vi "CRYUpdate Repeat State.vi"(0 "destination Index1":i32, 1 "fOption":bool, 5 "destination Index2":i32, 7 "My Index":i32, 9 "Start":dbl format="%#_5g", 11 "Increment":dbl, 12 "Count":i32, 13 "VI No":i32) -> (4 "fResult":bool)   [LabVIEW 2013]
uses:
  CRYProject Editor Global.vi
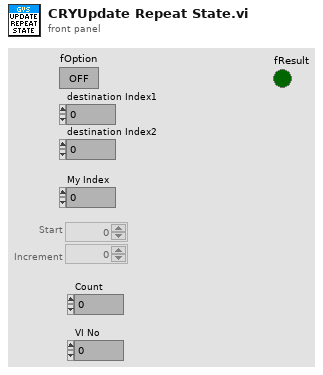
[diagram p1: front panel]
types:
  T1 = enum16{"OK", "Yes", "YesNo", "YesNoCancel", "ReplaceAppend"}
  T2 = typedef "CRYTS.ctl" = cluster{"No.TS":u16, "TS File Path":path, "TS Name":string, "EditStepName":string, "Steps":T3[], "New State":bool, "Change State":bool, "Flattened CurveLib Data":string, "Document Data":string, "EditStepNo":u16, "Operator Start File":string, "Sequence Type":string, "Sequence Language":string}
  T3 = typedef "CRYStep.ctl" = cluster{"No.VI":i32, "Category":string, "StepName":string, "Seq setup flattened":string, "Comment":string, "Steps config.":bool[], "Jump config":i32[], "Start":dbl, "Increment":dbl, "Name":string, "Unit":string, "Y data":u16, "Y prefix":string, "Y dB ref":dbl, "Y unit":string, "Repeat State Array":cluster{"Start":dbl, "Increment":dbl, "Count":i32, "Num":i32}[]}
  T4 = cluster{"Start":dbl, "Increment":dbl, "Count":i32, "Num":i32}[]
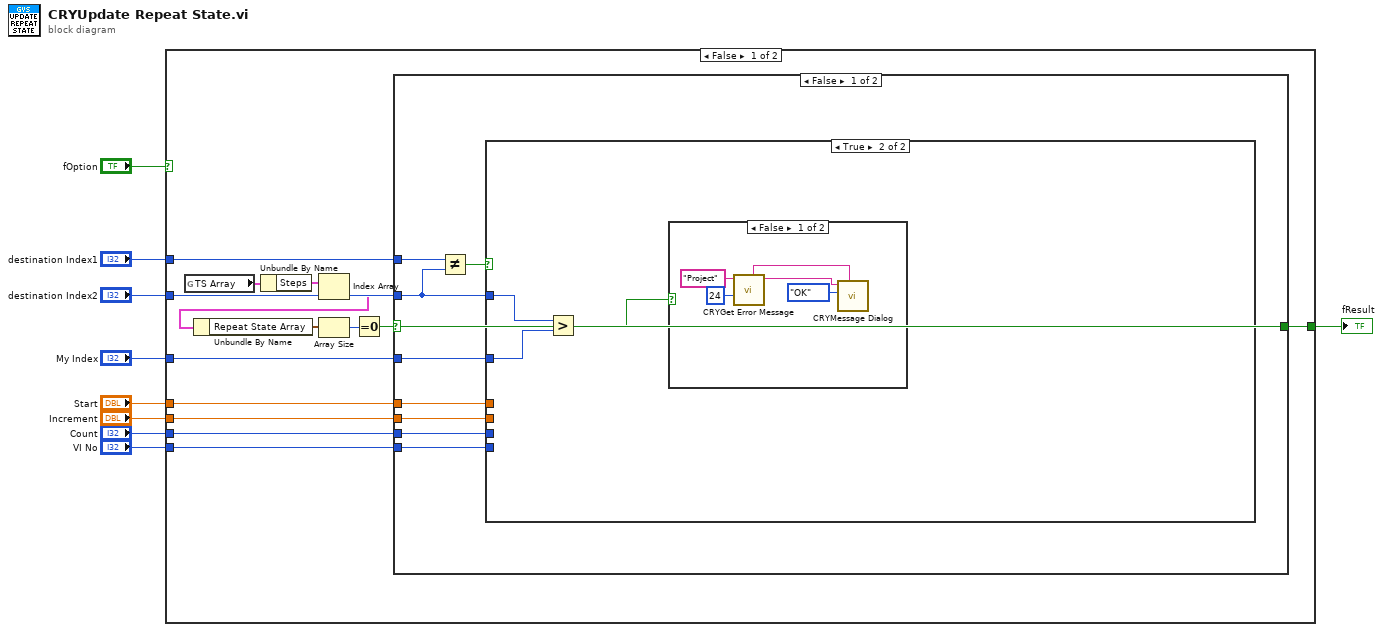
[diagram p0: block diagram]
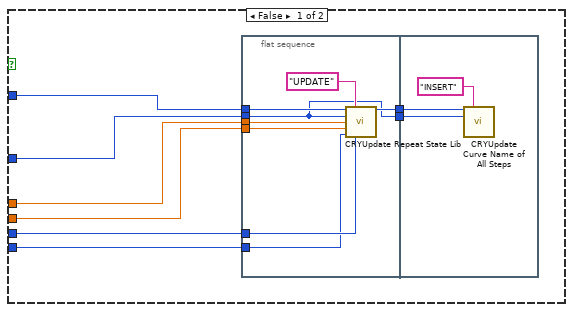
[diagram p2: hidden frame]
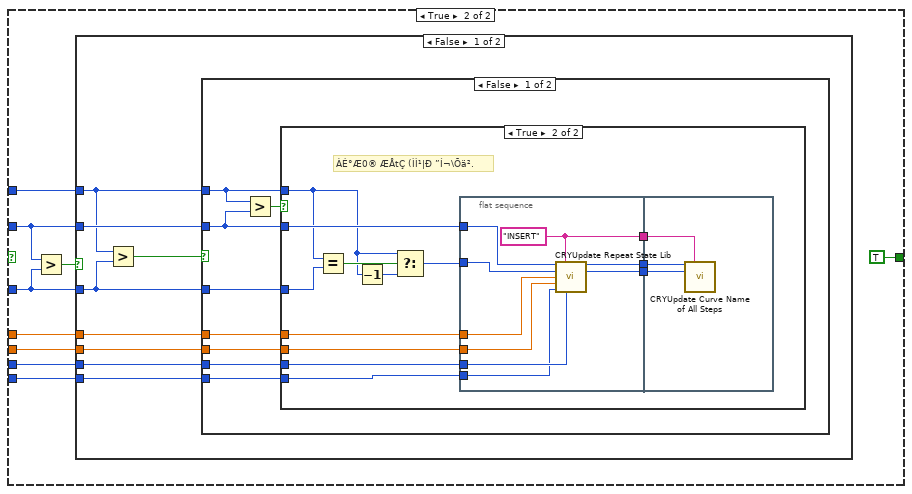
[diagram p4: hidden frame]
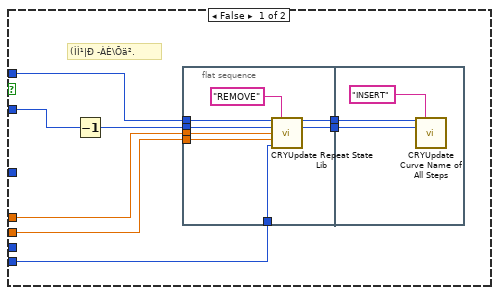
[diagram p5: hidden frame]
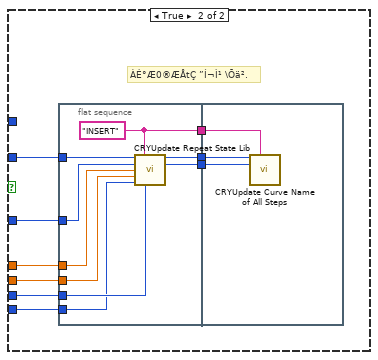
[diagram p6: hidden frame]
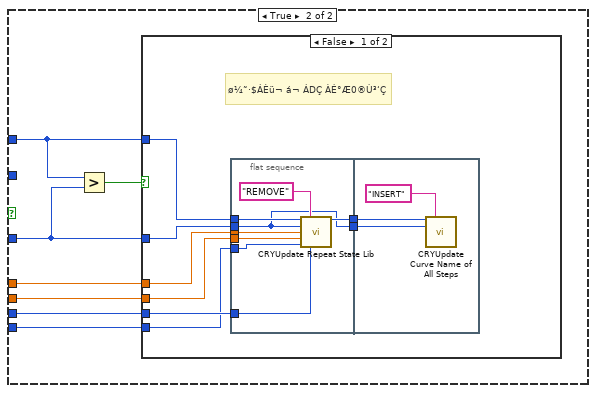
[diagram p7: hidden frame]
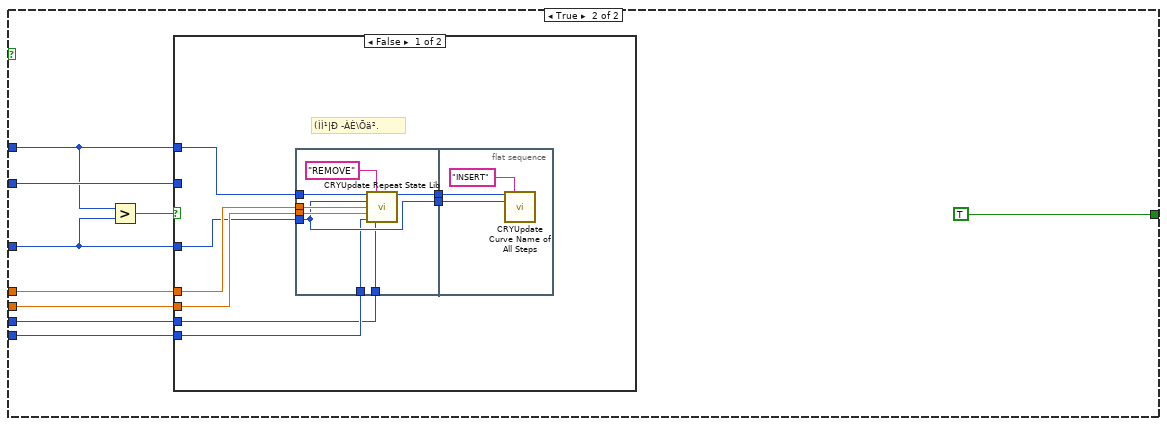
[diagram p9: hidden frame]
diagram:
  n1 = case shown="False" "fOption" {
    tunnel: [w23 TRUE] -> w9
    tunnel: "destination Index2" -> [w22 w175]
    tunnel: "My Index" -> [w21 w174]
    tunnel: "destination Index1" -> [w20 w173]
    tunnel: "Start" -> [w13 w172]
    tunnel: "Increment" -> [w12 w171]
    tunnel: "Count" -> [w11 w170]
    tunnel: "VI No" -> [w10 w168]
    frame False {
      n2 = global read "CRYProject Editor Global.vi" "TS Array"() -> (w19:T2)
      n3 = Unbundle By Name(w19) -> ("Steps"=w18:T3[])
      n4 = Index Array(array=w18, index=w22) -> (element=w17:T3)
      n5 = Unbundle By Name(w17) -> ("Repeat State Array"=w16:T4)
      n6 = Array Size(array=w16) -> (size(s)=w15:i32)
      n7 = Equal To 0?(x=w15) -> (x = 0?=w14:bool)
      n8 = case shown="False" w14 {
        selector: w14 -> [w32 _]
        tunnel: [w32 TRUE] -> w23
        tunnel: w21 -> [w28 w64]
        tunnel: w22 -> [w29 w63]
        tunnel: w20 -> [w31 w65]
        tunnel: w13 -> [w27 w62]
        tunnel: w12 -> [w26 w61]
        tunnel: w11 -> [w25 w60]
        tunnel: w10 -> [w24 w59]
        frame False {
          n9 = Not Equal?(x=w31, y=w29) -> (x != y?=w30:bool)
          n10 = case shown="True" w30 {
            tunnel: w29 -> [w40 w53]
            tunnel: w28 -> [w39 w52]
            tunnel: w27 -> [w38 _]
            tunnel: w26 -> [w37 _]
            tunnel: w25 -> [w36 _]
            tunnel: w24 -> [w33 _]
            frame False {
              n11 = flat-sequence {
                tunnel: w40 -> [w43]
                tunnel: w39 -> [w42]
                tunnel: w38 -> [w46]
                tunnel: w37 -> [w45]
                tunnel: w36 -> [w44]
                tunnel: [w43] -> w35
                tunnel: [w42] -> w34
                tunnel: w33 -> [w41]
                tunnel: w35 -> [w49]
                tunnel: w34 -> [w48]
                frame #0 {
                  n12 = call "CRYUpdate Repeat State Lib.vi"("Start Index"=w43, "sOption"="UPDATE", "End Index"=w42, "Start"=w46, "Increment"=w45, "Num"=w41, "Count"=w44) -> ()  [unwired: 9 in]
                }
                frame #1 {
                  n13 = call "CRYUpdate Curve Name of All Steps.vi"("Start Index"=w49, "sOption"="INSERT", "End Index"=w48) -> ()  [unwired: 13 in]
                }
              }
            }
            frame True {
              n14 = Greater?(x=w53, y=w52) -> (0:w51:bool)
              n15 = case shown="False" w51 {
                frame False {
                  n16 = call "CRYGet Error Message.vi"("Error No"=24, "Kind"="Project") -> ("Message"=w58:string, "Window Title"=w54:string)  [unwired: 4 in, 4 out]
                  n17 = call "CRYMessage Dialog.vi"("Window Title"=w54, "YesNoCancel"=T1."OK", "Message Content"=w58) -> ()  [unwired: 7 in, 2 out]
                }
                frame True {
                }
              }
            }
          }
        }
        frame True {
          n18 = Greater?(x=w63, y=w64) -> (0:w67:bool)
          n19 = case shown="False" w67 {
            tunnel: w65 -> [w73 w148]
            tunnel: w64 -> [w72 w147]
            tunnel: w63 -> [w74 _]
            tunnel: w62 -> [w71 w146]
            tunnel: w61 -> [w70 w145]
            tunnel: w60 -> [w69 w144]
            tunnel: w59 -> [w68 w143]
            frame False {
              n20 = Greater?(x=w73, y=w72) -> (0:w75:bool)
              n21 = case shown="False" w75 {
                tunnel: w74 -> [w82 w132]
                tunnel: w73 -> [w81 _]
                tunnel: w72 -> [w77 w128]
                tunnel: w71 -> [w80 w131]
                tunnel: w70 -> [w79 w130]
                tunnel: w69 -> [w78 w129]
                tunnel: w68 -> [w76 w124]
                frame False {
                  n22 = Greater?(x=w81, y=w82) -> (0:w83:bool)
                  n23 = case shown="True" w83 {
                    tunnel: w82 -> [w90 w113]
                    tunnel: w81 -> [w91 w107]
                    tunnel: w80 -> [w88 w112]
                    tunnel: w79 -> [w87 w111]
                    tunnel: w78 -> [_ w110]
                    tunnel: w77 -> [_ w109]
                    tunnel: w76 -> [w84 w101]
                    frame False {
                      # "(ÌÌ¹|Ð ­ÀÈ\\Õä²."
                      n24 = Decrement(x=w90) -> (x-1=w89:i32)
                      n25 = flat-sequence {
                        tunnel: w91 -> [w94]
                        tunnel: w89 -> [w93]
                        tunnel: w88 -> [w97]
                        tunnel: w87 -> [w96]
                        tunnel: [w94] -> w86
                        tunnel: [w93] -> w85
                        tunnel: w84 -> [w92]
                        tunnel: w86 -> [w100]
                        tunnel: w85 -> [w99]
                        frame #0 {
                          n26 = call "CRYUpdate Repeat State Lib.vi"("Start Index"=w94, "sOption"="REMOVE", "End Index"=w93, "Start"=w97, "Increment"=w96, "Num"=w92) -> ()  [unwired: 10 in]
                        }
                        frame #1 {
                          n27 = call "CRYUpdate Curve Name of All Steps.vi"("Start Index"=w100, "sOption"="INSERT", "End Index"=w99) -> ()  [unwired: 13 in]
                        }
                      }
                    }
                    frame True {
                      # "ÀÉ°Æ0® ÆÅtÇ (ÌÌ¹|Ð ”Í¬\\Õä²."
                      n28 = Equal?(x=w107, y=w109) -> (x = y?=w108:bool)
                      n29 = Decrement(x=w107) -> (x-1=w106:i32)
                      n30 = Select(t=w107, s=w108, f=w106) -> (s? t:f=w105:i32)
                      n31 = flat-sequence {
                        tunnel: w113 -> [w116]
                        tunnel: w112 -> [w120]
                        tunnel: w111 -> [w119]
                        tunnel: w110 -> [w118]
                        tunnel: w105 -> [w115]
                        tunnel: [w117] -> w104
                        tunnel: [w116] -> w103
                        tunnel: [w115] -> w102
                        tunnel: w101 -> [w114]
                        tunnel: w104 -> [w123]
                        tunnel: w103 -> [w122]
                        tunnel: w102 -> [w121]
                        frame #0 {
                          w117 = "INSERT" ("sOption")
                          n32 = call "CRYUpdate Repeat State Lib.vi"("Start Index"=w116, "sOption"=w117, "End Index"=w115, "Start"=w120, "Increment"=w119, "Num"=w114, "Count"=w118) -> ()  [unwired: 9 in]
                        }
                        frame #1 {
                          n33 = call "CRYUpdate Curve Name of All Steps.vi"("Start Index"=w122, "sOption"=w123, "End Index"=w121) -> ()  [unwired: 13 in]
                        }
                      }
                    }
                  }
                }
                frame True {
                  # "ÀÉ°Æ0®ÆÅtÇ ”Í¬Ì¹ \\Õä²."
                  n34 = flat-sequence {
                    tunnel: w132 -> [w135]
                    tunnel: w131 -> [w139]
                    tunnel: w130 -> [w138]
                    tunnel: w129 -> [w137]
                    tunnel: w128 -> [w134]
                    tunnel: [w136] -> w127
                    tunnel: [w135] -> w126
                    tunnel: [w134] -> w125
                    tunnel: w124 -> [w133]
                    tunnel: w127 -> [w142]
                    tunnel: w126 -> [w141]
                    tunnel: w125 -> [w140]
                    frame #0 {
                      w136 = "INSERT" ("sOption")
                      n35 = call "CRYUpdate Repeat State Lib.vi"("Start Index"=w135, "sOption"=w136, "End Index"=w134, "Start"=w139, "Increment"=w138, "Num"=w133, "Count"=w137) -> ()  [unwired: 9 in]
                    }
                    frame #1 {
                      n36 = call "CRYUpdate Curve Name of All Steps.vi"("Start Index"=w141, "sOption"=w142, "End Index"=w140) -> ()  [unwired: 13 in]
                    }
                  }
                }
              }
            }
            frame True {
              n37 = Greater?(x=w148, y=w147) -> (0:w149:bool)
              n38 = case shown="False" w149 {
                tunnel: w148 -> [w157 _]
                tunnel: w147 -> [w153 _]
                tunnel: w146 -> [w156 _]
                tunnel: w145 -> [w155 _]
                tunnel: w144 -> [w154 _]
                tunnel: w143 -> [w150 _]
                frame False {
                  # "ø¼˜·$ÁÈü¬ á¬ ÁDÇ ÀÉ°Æ0®Ù³‘Ç"
                  n39 = flat-sequence {
                    tunnel: w157 -> [w160]
                    tunnel: w156 -> [w164]
                    tunnel: w155 -> [w163]
                    tunnel: w154 -> [w162]
                    tunnel: w153 -> [w159]
                    tunnel: [w160] -> w152
                    tunnel: [w159] -> w151
                    tunnel: w150 -> [w158]
                    tunnel: w152 -> [w167]
                    tunnel: w151 -> [w166]
                    frame #0 {
                      n40 = call "CRYUpdate Repeat State Lib.vi"("Start Index"=w160, "sOption"="REMOVE", "End Index"=w159, "Start"=w164, "Increment"=w163, "Num"=w158, "Count"=w162) -> ()  [unwired: 9 in]
                    }
                    frame #1 {
                      n41 = call "CRYUpdate Curve Name of All Steps.vi"("Start Index"=w167, "sOption"="INSERT", "End Index"=w166) -> ()  [unwired: 13 in]
                    }
                  }
                }
                frame True {
                  # "DÅ4»ƒ¬Ä³ XÕÀÉ JÅ”²ä²"
                }
              }
            }
          }
        }
      }
    }
    frame True {
      n42 = Greater?(x=w173, y=w174) -> (0:w169:bool)
      n43 = case shown="False" w169 {
        tunnel: w175 -> [_ _]
        tunnel: w173 -> [w184 _]
        tunnel: w174 -> [w181 _]
        tunnel: w172 -> [w183 _]
        tunnel: w171 -> [w182 _]
        tunnel: w170 -> [w177 _]
        tunnel: w168 -> [w178 _]
        frame False {
          # "(ÌÌ¹|Ð ­ÀÈ\\Õä²."
          n44 = flat-sequence {
            tunnel: w184 -> [w188]
            tunnel: w183 -> [w191]
            tunnel: w182 -> [w190]
            tunnel: w181 -> [w187]
            tunnel: [w188] -> w180
            tunnel: [w187] -> w179
            tunnel: w178 -> [w186]
            tunnel: w177 -> [w185]
            tunnel: w180 -> [w194]
            tunnel: w179 -> [w193]
            frame #0 {
              n45 = call "CRYUpdate Repeat State Lib.vi"("Start Index"=w188, "sOption"="REMOVE", "End Index"=w187, "Start"=w191, "Increment"=w190, "Num"=w186, "Count"=w185) -> ()  [unwired: 9 in]
            }
            frame #1 {
              n46 = call "CRYUpdate Curve Name of All Steps.vi"("Start Index"=w194, "sOption"="INSERT", "End Index"=w193) -> ()  [unwired: 13 in]
            }
          }
        }
        frame True {
        }
      }
    }
  }
  "fResult" <- w9
